vi "SCD - Externally Triggered Image Acquisition - Basic Building Block Using Queues.vi"(0 "FPS":dbl=10.0 format="%0.2p", 1 "LCVR Voltages":dbl[][](array[numeric]), 5 "Modulation Cycles":i32=1 min=1 max=30 step=1, 9 "Headers In":T4[](array[typedef])=[{"Wavelength (nm)"=530.15, "Exposure (s)"=0.05, "Tuning Delay (ms)"=1000.0, "Beam Type (-1/1)"=1.0, "Tuning Voltages"=[1.111, 2.222, 3.333, 4.444], "Observer"="observer", "Light Shapping Diffuser"=enum."In Beam", "Comment"="", "Data Type"=9, "Mod Cycles"=0, "SCD Calibration Optics"=enum."1 - Polarizer @0, I+Q", "SCD Emission Line Filter"=enum."1-557.6nm", "Cookbook"="", "COMP-S Calibration Wheel"=enum."Dark", "COMP-S Andover Filter Wheel"=enum."530.3nm/HWB 0.34nm (Fe XIV)", "FOV Rotation (deg)"=66.0, "Objective Lens Position (mm)"=0.0, "Occulter size"=0.0, "Time End"=timestamp(3382374145.421875 s since 1904-01-01), "Acc Exposure (s)"=0.0, "Time Stamp Array"=[], "Camera Serial Number"=[], "Camera Temp"=[], "Camera PI (mm)"=[0.0, 0.0, 0.0], "Time Start"=timestamp(3382374145.421875 s since 1904-01-01), "Peripherals"={"ILX controler"=FALSE, "Zone temperatures"=FALSE, "Andor"=FALSE, "Andor 2"=FALSE, "PI Stage"=FALSE, "AISAS mechanisms"=FALSE, "AISAS Mech.lvclass"=refnum, "Zone temp ref"=variant, "FW"=FALSE}}] {"Camera PI (mm)" format="%_3g"; "Acc Exposure (s)" format="%^.3g"; "Occulter size" format="%.2f"; "Objective Lens Position (mm)" min=70.0 max=152.0 format="%.2f"; "FOV Rotation (deg)" format="%.1f"; "Data Type" items=["LIVE", "DARK", "FLAT", "CALI", "OBSE", "ABSO", "AURE", "TARG", "OBJE", "HOLE", "OREX", "THRO", "CHIP"]; "Exposure (s)" format="%^.3g"; "Wavelength (nm)" format="%_6g"}, 11 "error in":errorcluster, 12 "Neo Info":T2={"Handle"=104, "Pixel Encoding"="Mono16", "AOI Width"=2560, "AOI Height"=2160, "AOI Stride"=5136, "Image Bytes"=11098896, "Image Pixels"=5529600, "Row Readout Time"=9.371428571428572e-06, "Frame Readout Time"=0.010121142857142858, "Interframe Time"=8.434285714285715e-05, "Semaphore"=refnum, "SerialNumber"="SCC-02209", "Camera Model"="DC-152Q-C00-FI", "Controller ID"="3", "Firmware Version"="13.8.26.122", "Shutter"="Global", "Binning"=0, "Time at Synch"=timestamp(3029526000.379448 s since 1904-01-01), "Idx"=0} {"Time at Synch" format="%<%H:%M:%S>T"; "Interframe Time" format="%#_3g"; "Frame Readout Time" format="%_3g"; "Row Readout Time" format="%_3g"}, 14 "Timestamp at Synch":timestamp) -> (3 "FITS Path Out":path, 4 "Andor Handle Out":i32, 6 "Most Recent Image Accumulation (Modulation State A)":u32[][](graph), 10 "Headers Out":T4[](array[typedef]) {"Camera PI (mm)" format="%_3g"; "Acc Exposure (s)" format="%^.3g"; "Occulter size" format="%.2f"; "Objective Lens Position (mm)" min=70.0 max=152.0 format="%.2f"; "FOV Rotation (deg)" format="%.1f"; "Data Type" items=["LIVE", "DARK", "FLAT", "CALI", "OBSE", "ABSO", "AURE", "TARG", "OBJE", "HOLE", "OREX", "THRO", "CHIP"]; "Exposure (s)" format="%^.3g"; "Wavelength (nm)" format="%_6g"}, 15 "error out":errorcluster={"status"=FALSE, "code"=5000, "source"="AT Finalise Library A.vi\n\nSUCCESS"})   [LabVIEW 2014]
doc: "The LL Sequence VI acquires a sequence of images and displays them in an array of image controls using the low-level acquisition VIs. A sequence is appropriate for applications that process multiple images. You can configure a sequence to acquire every frame or to skip a variable number of frames between each image.\n\nTop Level Code Overview\n1) Initialize Camera (Global Shutter, High Well, Low Noise, exposure time, etc.)\n2) Create a buffer set equal in size to the # of trigger pulses (e.g. 100) which is the same as the # of expected images \n3) Start the camera acquisition THEN start the DAQmx task (use merge error cluster to gurantee this)"
uses:
  <vilib>/DAQmx/configure/timing.llb/DAQmx Timing (Use Waveform).vi
  <vilib>/DAQmx/create/channels.llb/DAQmx Create Channel (AO-Voltage-Basic).vi
  <vilib>/DAQmx/write.llb/DAQmx Write (Analog 1D Wfm NChan NSamp).vi
  <vilib>/Waveform/WDTOps.llb/WDT Waveform Duration DBL.vi
  Controls/SCD - Calibration Optics Filter Wheel.ctl
  AISAS/Controls/Diffuser.ctl
  Controls/SCD - FITS Cluster.ctl
  Camera/Andor Neo Info.ctl
  Controls/SCD - EDT - Emission Line Filter Wheel.ctl
  Controls/CoMP-S Controls/Polarization Optics Filter Wheel.ctl
  Controls/CoMP-S Controls/Emission Line Filter Wheel.ctl
  AISAS/Controls/focus.ctl
  AISAS/Mech/AISAS Mech.lvclass
  Controls/peripherals.ctl
panel:
  in  "Tab Control":T1(tab)
  out "# images to acquire":i32
  out "SCD Waveforms (Graph)":waveform(dbl)[](graph)
  out "Image Acquisition Started":bool
  out "PixelData [U16]":u16[](array[numeric])
  out "ByteData [U8]":u8[](array[numeric])
  out "Andor Handle In":i32=104
  in  "image pointers":u64[](array[numeric])
  in  "imageNo":i32
  in  "count":i32
  in  "physical channels":tag="PXI-6733/ao0:7"
  out "Acquisition Estimate (s)":dbl=0.6002500000000001 format="%0.2f"
  out "# Wavelengths":i32=1
  out "Exposure Get (s)":dbl=0.09
  out "Image Acq (s)":dbl(slide)=4151.832132564842
  out "# elements in queue":i32
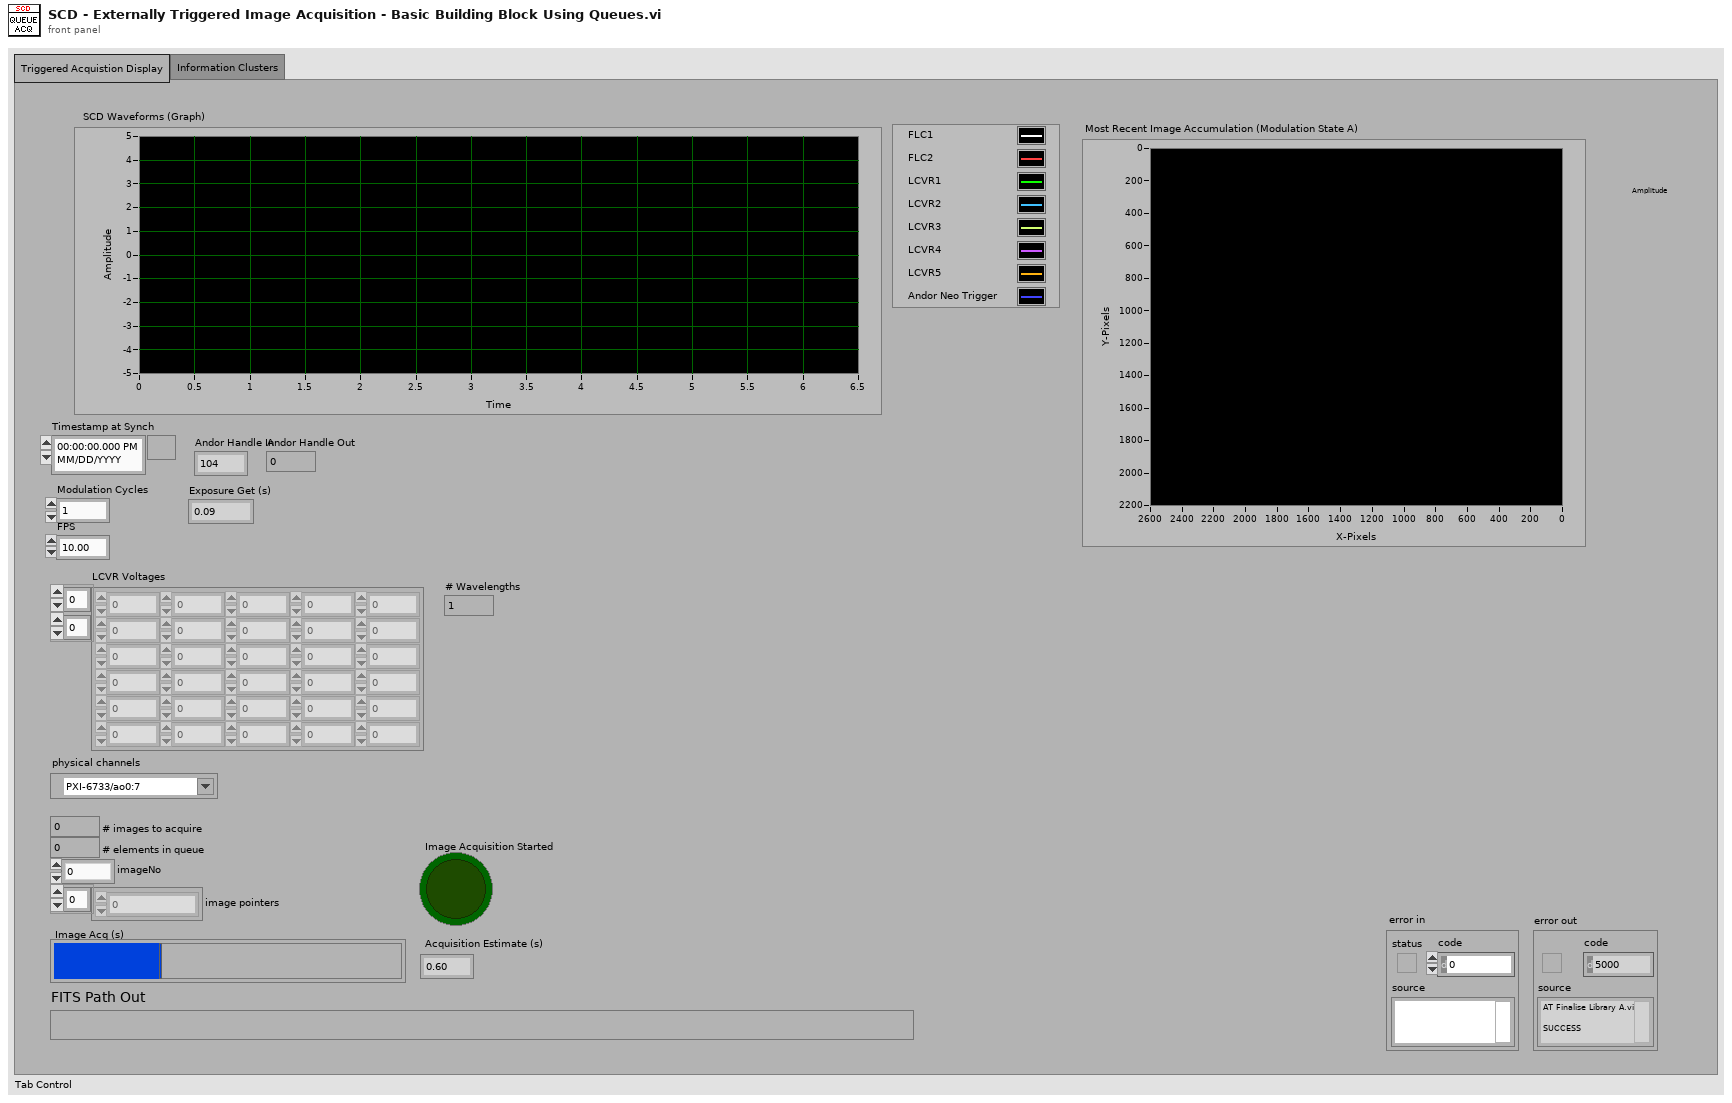
[diagram p1: front panel]
types:
  T1 = enum32{"Triggered Acquistion Display", "Information Clusters"}
  T2 = typedef "Andor Neo Info.ctl" = cluster{"Handle":i32, "Pixel Encoding":string, "AOI Width":i64, "AOI Height":i64, "AOI Stride":i64, "Image Bytes":i64, "Image Pixels":i64, "Row Readout Time":dbl, "Frame Readout Time":dbl, "Interframe Time":dbl, "Semaphore":T3, "SerialNumber":string, "Camera Model":string, "Controller ID":string, "Firmware Version":string, "Shutter":string, "Binning":u8, "Time at Synch":timestamp, "Idx":i32}
  T3 = typedef "Semaphore RefNum" = refnum<k1>
  T4 = typedef "SCD - FITS Cluster.ctl" = cluster{"Wavelength (nm)":dbl, "Exposure (s)":dbl, "Tuning Delay (ms)":dbl, "Beam Type (-1/1)":dbl, "Tuning Voltages":dbl[], "Observer":string, "Light Shapping Diffuser":T5, "Comment":string, "Data Type":u16, "Mod Cycles":u16, "SCD Calibration Optics":T6, "SCD Emission Line Filter":T7, "Cookbook":string, "COMP-S Calibration Wheel":T8, "COMP-S Andover Filter Wheel":T9, "FOV Rotation (deg)":dbl, "Objective Lens Position (mm)":T10, "Occulter size":dbl, "Time End":timestamp, "Acc Exposure (s)":dbl, "Time Stamp Array":timestamp[], "Camera Serial Number":string[], "Camera Temp":dbl[], "Camera PI (mm)":dbl[], "Time Start":timestamp, "Peripherals":T11}
  T5 = typedef "Diffuser.ctl" = enum16{"Out of Beam", "In Beam"}
  T6 = typedef "SCD - Calibration Optics Filter Wheel.ctl" = enum16{"1 - Polarizer @0, I+Q", "2 - Polarizer @90, I-Q", "3 - Polarizer @45, I+U", "4 - Polarizer @135, I-U", "5 - Polarizer @0, Retarder @45, I+V", "6 - Polarizer @0, Retarder @135, I-V", "7 - Dark", "8 - Clear", "9 - N/A"}
  T7 = typedef "SCD - EDT - Emission Line Filter Wheel.ctl" = enum16{"1-557.6nm", "2-587.6nm", "3-589.6nm", "4-630.2nm", "5-656.4nm", "6-849.8nm", "7-854.2nm", "8-866.2nm", "9-1083.0nm"}
  T8 = typedef "Polarization Optics Filter Wheel.ctl" = enum16{"Dark", "Clear", "Exchange Lens", "Polarizer @0, I+Q", "Polarizer @90, I-Q", "Polarizer @45, I+U", "Polarizer @135, I-U", "Polarizer @0, Retarder @45, I+V", "Polarizer @0, Retarder @135, I-V"}
  T9 = typedef "Emission Line Filter Wheel.ctl" = enum16{"530.3nm/HWB 0.34nm (Fe XIV)", "587.6nm/HBW 0.44nm (He I D3)", "637.5nm/HBW 0.53nm (Fe X)", "656.3nm/HBW 0.57nm (H-Alpha)", "789.2nm/HBW 0.85nm (Fe XI)", "854.2nm/HBW 1.01nm (Ca I)", "1074.7nm/HBW 2.34nm (Fe XIII)", "1079.8nm/HBW 1.64nm (Fe XIII)", "1083.0nm/HBW 1.66nm (He I)"}
  T10 = typedef "focus.ctl" = dbl
  T11 = typedef "peripherals.ctl" = cluster{"ILX controler":bool, "Zone temperatures":bool, "Andor":bool, "Andor 2":bool, "PI Stage":bool, "AISAS mechanisms":bool, "AISAS Mech.lvclass":refnum<class "AISAS Mech.lvclass">, "Zone temp ref":variant, "FW":bool}
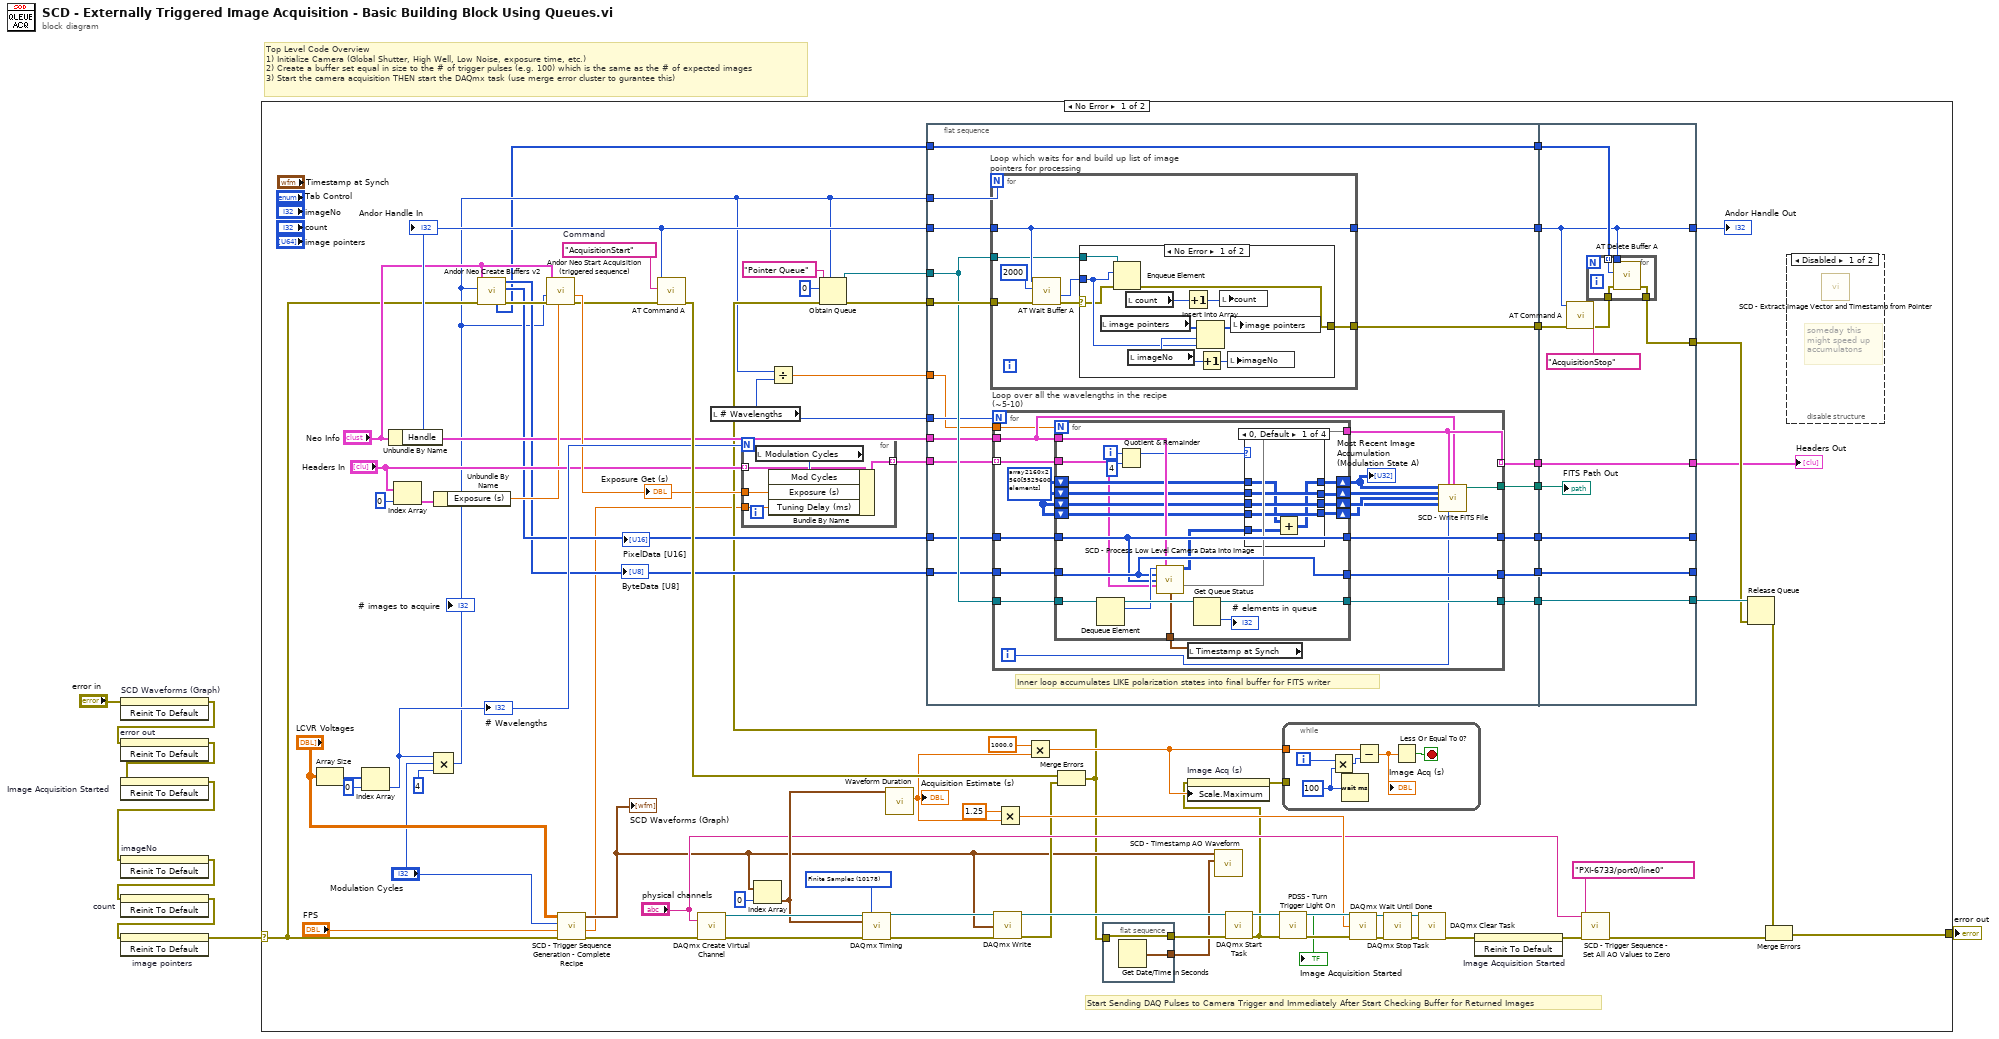
[diagram p0: block diagram]
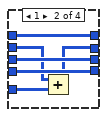
[diagram p3: hidden frame]
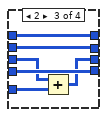
[diagram p4: hidden frame]
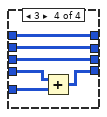
[diagram p5: hidden frame]
diagram:
  # "Top Level Code Overview\n1) Initialize Camera (Global Shutter, High Well, Low Noise, exposure time, etc.)\n2) Create a buffer set equal in size to the # of trigger pulses (e.g. 100) which is the same as the # of expected images \n3) Start the camera acquisition THEN start the DAQmx task (use merge error cluster to gurantee this)"
  n1 = invoke on="SCD Waveforms (Graph)" class="WFGraph (strict)" method="Reinit To Default"(error in="error in") -> (error out=w6:errorcluster)  [unwired: 2 in, 2 out]
  n2 = invoke on="error out" class="Clust (strict)" method="Reinit To Default"(error in=w6) -> (error out=w5:errorcluster)  [unwired: 2 in, 2 out]
  n3 = invoke on="Image Acquisition Started" class="Bool (strict)" method="Reinit To Default"(error in=w5) -> (error out=w1:errorcluster)  [unwired: 2 in, 2 out]
  n4 = invoke on="imageNo" class="DigNum (strict)" method="Reinit To Default"(error in=w1) -> (error out=w4:errorcluster)  [unwired: 2 in, 2 out]
  n5 = invoke on="count" class="DigNum (strict)" method="Reinit To Default"(error in=w4) -> (error out=w3:errorcluster)  [unwired: 2 in, 2 out]
  n6 = invoke on="image pointers" class="Arr (strict)" method="Reinit To Default"(error in=w3) -> (error out=w2:errorcluster)  [unwired: 2 in, 2 out]
  n7 = case shown="No Error" w2 {
    selector: w2 -> [w22 w216]
    tunnel: [w55 w216] -> w8
    frame No Error {
      w60 = "AcquisitionStart"  # Command
      w86 = 10178 items=["Finite Samples"=10178, "Continuous Samples"=10123] ("sample mode")
      # "Start Sending DAQ Pulses to Camera Trigger and Immediately After Start Checking Buffer for Returned Images"
      n8 = Array Size(array="LCVR Voltages") -> (size(s)=w68:i32[])
      n9 = Index Array(array=w68, index=0) -> (element=w47:i32)
      "# Wavelengths" <- w47
      n10 = Unbundle By Name("Neo Info") -> ("Handle"=w54:i32)
      "Andor Handle In" <- w54
      n11 = Index Array(array="Headers In", index=0) -> (element=w42:T4)
      n12 = Unbundle By Name(w42) -> ("Exposure (s)"=w41:dbl)
      n13 = Compound Arithmetic op=MULTIPLY(w47, "Modulation Cycles", 4 ("value")) -> (w12:i32)
      "# images to acquire" <- w12
      n14 = call "Andor Neo Create Buffers v2.vi"("error in"=w22, "Number of Buffers"=w12, "Camera Info"="Neo Info") -> ("error out"=w53:errorcluster, "PixelData"=w35:i64[], "ByteData"=w33:u8[], "Array of Buffers"=w11:u64[])  [unwired: 5 in]
      "ByteData [U8]" <- w33
      "PixelData [U16]" <- w35
      n15 = call "Andor Neo Start Acquisition (triggered sequence).vi"("Exposure Set (s)"=w41, "error in"=w53, "Frames"=w12, "Camera Info"="Neo Info") -> ("error out"=w39:errorcluster, "Exposure Get (s)"=w45:dbl)  [unwired: 6 in]
      "Exposure Get (s)" <- w45
      n16 = call "SCD - Trigger Sequence Generation - Complete Recipe.vi"("error in"=w22, "FPS"="FPS", "Modulation Cycles\nAt Each Wavelength"="Modulation Cycles", "LCVR Voltages"="LCVR Voltages") -> ("error out"=w76:errorcluster, "LCVR Relaxtion Time"=w9:dbl, "SCD Waveforms (Graph)"=w48:waveform(dbl)[])  [unwired: 5 in]
      "SCD Waveforms (Graph)" <- w48
      n17 = call <userlib>:"AT Command A.vi"("error in (no error)"=w39, "Feature"=w60, "Handle"=w54) -> ("error out"=w52:errorcluster)  [unwired: 7 in, 1 out]
      n18 = call-poly <vilib>:"DAQmx Create Virtual Channel.vi"("physical channels"="physical channels", "error in"=w76) -> ("task out"=w83:refnum<k21>, "error out"=w84:errorcluster)  [unwired: 12 in]
      n19 = local read "# Wavelengths"() -> (w20:i32)
      n20 = for {
        N: w47 -> [_]
        tunnel: [w96] -> w37 mode=indexing
        tunnel: w45 -> [w95]
        tunnel: "Headers In" -> [w94] mode=indexing
        tunnel: w9 -> [w93]
        n21 = local read "Modulation Cycles"() -> (w97:i32)
        n22 = Bundle By Name(cluster=w94, "Mod Cycles"=w97, "Exposure (s)"=w95, "Tuning Delay (ms)"=w93) -> (w96:T4)
      }
      n23 = Index Array(array=w48, index=0) -> (element=w73:waveform(dbl))
      n24 = Divide(x=w12, y=w20) -> (x/y=w21:dbl)
      n25 = call-poly <vilib>:"DAQmx Timing.vi"("task/channels in"=w83, "sample mode"=w86, "waveform"=w73, "error in"=w84) -> ("task out"=w74:refnum<k21>, "error out"=w75:errorcluster)  [unwired: 10 in]
      n26 = call-poly <vilib>:"Waveform Duration.vi"("waveform in"=w73) -> ("duration"=w25:dbl)  [unwired: 8 in, 2 out]
      "Acquisition Estimate (s)" <- w25
      n27 = flat-sequence {
        tunnel: w30 -> [w117]
        tunnel: w12 -> [w105]
        tunnel: w54 -> [w116]
        tunnel: [w115] -> w59
        tunnel: [w114] -> w58
        tunnel: "Neo Info" -> [w106]
        tunnel: w37 -> [w108]
        tunnel: [w107] -> w36
        tunnel: w35 -> [w109]
        tunnel: [w104] -> w34
        tunnel: w33 -> [w112]
        tunnel: [w110] -> w32
        tunnel: w29 -> [w113]
        tunnel: [w111] -> w27
        tunnel: w21 -> [w100]
        tunnel: w20 -> [w103]
        tunnel: [w102] -> w19
        tunnel: w11 -> [w101]
        tunnel: [w101] -> w10
        tunnel: w59 -> [w204]
        tunnel: w58 -> [w210]
        tunnel: [w204] -> w51
        tunnel: [w202] -> w16
        tunnel: [w209] -> w15
        tunnel: w36 -> [w209]
        tunnel: [w208] -> _
        tunnel: w34 -> [w208]
        tunnel: [w207] -> _
        tunnel: w32 -> [w207]
        tunnel: w27 -> [w206]
        tunnel: [w206] -> w26
        tunnel: w19 -> [w201]
        tunnel: w10 -> [w205]
        frame #0 {
          # "Inner loop accumulates LIKE polarization states into final buffer for FITS writer"
          n28 = for "Loop which waits for and build up list of image pointers for processing" {
            N: w105 -> [_]
            tunnel: w116 -> [w186]
            tunnel: w117 -> [w188]
            tunnel: [w186] -> w115
            tunnel: [w184] -> w114
            tunnel: w113 -> [w183]
            n29 = call <userlib>:"AT Wait Buffer A.vi"("error in (no error)"=w188, "Timeout"=u32 2000, "Handle"=w186) -> ("error out"=w185:errorcluster, "Output buffer"=w187:u64)  [unwired: 5 in, 2 out]
            n30 = case shown="No Error" w185 {
              selector: w185 -> [w191 w200]
              tunnel: w187 -> [w193 _]
              tunnel: [w190 w200] -> w184
              tunnel: w183 -> [w192 _]
              frame No Error {
                n31 = local read "image pointers"() -> (w197:u64[])
                n32 = Enqueue Element(queue=w192, element=w193, error in (no error)=w191) -> (error out=w190:errorcluster)  [unwired: 1 in, 2 out]
                n33 = local read "count"() -> (w199:i32)
                n34 = local read "imageNo"() -> (w194:i32)
                n35 = Increment(x=w199) -> (x+1=w198:i32)
                n36 = Insert Into Array(array=w197, index=w194, new element=w193) -> (w196:u64[])
                n37 = Increment(x=w194) -> (x+1=w195:i32)
                n38 = local write "count"(w198) -> ()
                n39 = local write "imageNo"(w195) -> ()
                n40 = local write "image pointers"(w196) -> ()
              }
              frame Error {
              }
            }
          }
          n41 = for "Loop over all the wavelengths in the recipe (~5-10)" {
            N: w103 -> [_]
            tunnel: w113 -> [w135]
            tunnel: w112 -> [w134]
            tunnel: [w133] -> w111
            tunnel: [w132] -> w110
            tunnel: w109 -> [w131]
            tunnel: w108 -> [w130] mode=indexing
            tunnel: [w122] -> w107 mode=indexing
            tunnel: w106 -> [w120]
            tunnel: [w125] -> w104
            tunnel: [w124] -> w102
            tunnel: w100 -> [w119]
            i -> [w118]
            w129 = i32[][] array2160x2560[5529600 elements] ("2560x2160 Initialized Array")
            n42 = local read "Timestamp at Synch"() -> (w123:timestamp)
            n43 = for {
              N: w119 -> [_]
              tunnel: w135 -> [w158]
              tunnel: w134 -> [w155]
              tunnel: [w140] -> w133
              tunnel: [w155] -> w132
              tunnel: w131 -> [w154]
              tunnel: [w154] -> w125
              tunnel: w130 -> [w138]
              tunnel: [w137] -> w122
              tunnel: w120 -> [w153]
              shift-right: [w145] -> w121
              shift-left: w129 -> [w146]
              shift-right: [w144] -> w128
              shift-left: w129 -> [w147]
              shift-right: [w143] -> w127
              shift-left: w129 -> [w148]
              shift-right: [w142] -> w126
              shift-left: w129 -> [w149]
              tunnel: w123 -> [w136]
              i -> [w151]
              n44 = Dequeue Element(queue=w158) -> (queue out=w157:refnum<queue>, element=w156:u64)  [unwired: 2 in, 2 out]
              n45 = Quotient & Remainder(x=w151, y=4) -> (x-y*floor(x/y)=w150:i32)  [unwired: 1 out]
              n46 = call "SCD - Process Low Level Camera Data Into Image.vi"("Pointer In"=w156, "Neo Info"=w153, 2:w136, "ByteData (U8)"=w155, "PixelData (U16)"=w154, 9:w138) -> ("Image (I32)"=w141:u32[][], 10:w137)  [unwired: 6 in, 2 out]
              n47 = Get Queue Status(queue=w157) -> (queue out=w140:refnum<queue>, # elements in queue=→"# elements in queue":i32)  [unwired: 2 in, 6 out]
              n48 = case shown="0, Default" w150 {
                tunnel: w149 -> [w162 w169 w175 w178]
                tunnel: w148 -> [w163 w170 w172 w181]
                tunnel: w147 -> [w164 w166 w176 w182]
                tunnel: w146 -> [w160 w167 w173 w179]
                tunnel: [w159 w167 w173 w179] -> w145
                tunnel: [w164 w165 w176 w182] -> w144
                tunnel: [w163 w170 w171 w181] -> w143
                tunnel: [w162 w169 w175 w177] -> w142
                tunnel: w141 -> [w161 w168 w174 w180]
                frame 0, Default {
                  n49 = Add(x=w160, y=w161) -> (x+y=w159:u32[][])
                }
                frame 1 {
                  n50 = Add(x=w166, y=w168) -> (x+y=w165:u32[][])
                }
                frame 2 {
                  n51 = Add(x=w172, y=w174) -> (x+y=w171:u32[][])
                }
                frame 3 {
                  n52 = Add(x=w178, y=w180) -> (x+y=w177:u32[][])
                }
              }
            }
            "Most Recent Image Accumulation (Modulation State A)" <- w121
            n53 = call "SCD - Write FITS File.vi"("A"=w121, "FITS Header"=w122, "Neo Info"=w120, "B"=w128, "C"=w127, "D"=w126, "Image #"=w118) -> ("FITS Path Out"=w124:path)  [unwired: 6 in, 2 out]
          }
        }
        frame #1 {
          n54 = call <userlib>:"AT Command A.vi"("error in (no error)"=w210, "Feature"="AcquisitionStop" ("Command"), "Handle"=w204) -> ("error out"=w203:errorcluster)  [unwired: 7 in, 1 out]
          n55 = for {
            tunnel: w205 -> [w215] mode=indexing
            tunnel: w204 -> [w214]
            tunnel: w203 -> [w213]
            tunnel: [w212] -> w202
            n56 = call <userlib>:"AT Delete Buffer A.vi"("error in (no error)"=w213, "Buffer"=w215, "Handle"=w214) -> ("error out"=w212:errorcluster)  [unwired: 7 in, 1 out]
          }
          "FITS Path Out" <- w201
        }
      }
      n57 = call-poly <vilib>:"DAQmx Write.vi"("task/channels in"=w74, "data"=w48, "error in"=w75) -> ("task out"=w85:refnum<k21>, "error out"=w57:errorcluster)  [unwired: 10 in, 1 out]
      n58 = Multiply(x=1.25, y=w25) -> (x*y=w63:dbl)
      n59 = Multiply(x=1000.0, y=w25) -> (x*y=w23:dbl)
      n60 = Merge Errors(w52, w57) -> (w17:errorcluster)
      n61 = Obtain Queue(max queue size (-1, unlimited)=w12, name (unnamed)="Pointer Queue", element data type=u64 0 ("Output buffer"), error in (no error)=w17) -> (queue out=w29:refnum<queue>, error out=w30:errorcluster)  [unwired: 1 in, 1 out]
      n62 = flat-sequence {
        tunnel: [w99] -> w50
        tunnel: w17 -> [w99]
        tunnel: [w98] -> w49
        frame #0 {
          n63 = Get Date/Time In Seconds() -> (seconds since 1Jan1904=w98:timestamp)
        }
      }
      n64 = call "SCD - Timestamp AO Waveform.vi"("DAQ To"=w49, "SCD AO Waveforms"=w48) -> ()  [unwired: 8 in, 2 out]
      n65 = call <vilib>:"DAQmx Start Task.vi"("task/channels in"=w85, "error in"=w50) -> ("task out"=w82:refnum<k21>, "error out"=w14:errorcluster)  [unwired: 12 in]
      n66 = property on="Image Acq (s)" class="Slide (strict)"(error in=w14, "Scale.Maximum"=w23) -> (error out=w13:errorcluster)  [unwired: 1 in, 1 out]
      n67 = call "PDSS - Turn Trigger Light On.vi"("error in (no error)"=w14) -> ("error out"=w71:errorcluster, "Trigger Started"=→"Image Acquisition Started":bool)  [unwired: 9 in]
      n68 = while {
        tunnel: w23 -> [w91]
        tunnel: w13 -> [_]
        i -> [w89]
        stop <- w90 stop-if-true
        w88 = u32 100 ("milliseconds to wait")
        n69 = Multiply(x=w89, y=w88) -> (x*y=w92:u32)
        n70 = Wait (ms)(milliseconds to wait=w88) -> ()  [unwired: 1 out]
        n71 = Subtract(x=w91, y=w92) -> (x-y=w87:dbl)
        "Image Acq (s)" <- w87
        n72 = Less Or Equal To 0?(x=w87) -> (x <= 0?=w90:bool)
      }
      n73 = call <vilib>:"DAQmx Wait Until Done.vi"("task/channels in"=w82, "timeout (sec)"=w63, "error in"=w71) -> ("task out"=w81:refnum<k21>, "error out"=w80:errorcluster)  [unwired: 11 in]
      n74 = call <vilib>:"DAQmx Stop Task.vi"("task/channels in"=w81, "error in"=w80) -> ("task out"=w79:refnum<k21>, "error out"=w78:errorcluster)  [unwired: 12 in]
      n75 = call <vilib>:"DAQmx Clear Task.vi"("task in"=w79, "error in"=w78) -> ("error out"=w65:errorcluster)  [unwired: 13 in]
      n76 = invoke on="Image Acquisition Started" class="Bool (strict)" method="Reinit To Default"(error in=w65) -> (error out=w64:errorcluster)  [unwired: 2 in, 2 out]
      n77 = call "SCD - Trigger Sequence - Set All AO Values to Zero.vi"("error in"=w64, "lines"=tag "PXI-6733/port0/line0", "physical channels"="physical channels") -> ("error out"=w56:errorcluster)  [unwired: 8 in]
      n78 = Release Queue(queue=w26, error in (no error)=w16) -> (error out=w18:errorcluster)  [unwired: 1 in, 2 out]
      n79 = Merge Errors(w18, w56) -> (w55:errorcluster)
      n80 = disable-structure shown="Disabled" {
        frame Disabled {
          # "someday this\nmight speed up\naccumulatons"
          n81 = call "SCD - Extract Image Vector and Timestamp from Pointer.vi"() -> ()  [unwired: 13 in, 3 out]
        }
        frame Enabled {
        }
      }
      "Andor Handle Out" <- w51
      "Headers Out" <- w15
    }
    frame Error {
    }
  }
  "error out" <- w8
